vi "Actuators.vi"() -> ()   [LabVIEW 2023]
panel:
  in  "main-fan-switch":bool
  in  "main-light-switch":bool
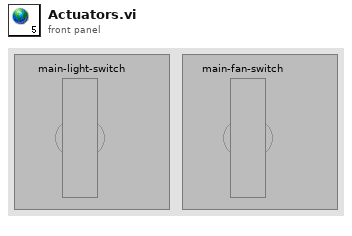
[diagram p1: front panel]
diagram:
